vi "UnusedVI.vi"(9 "Queue in":refnum<queue>, 10 "queue in":refnum<queue>, 11 "String in":refnum<vi>) -> (3 "current sensor line ASCII":string)   [LabVIEW 2013]
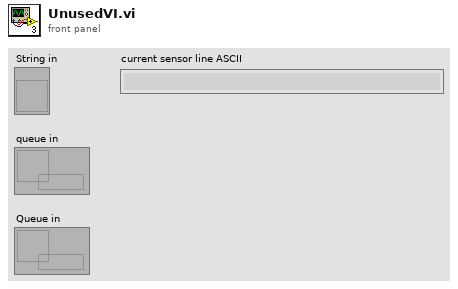
[diagram p1: front panel]
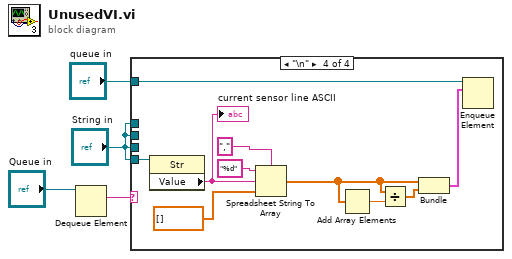
[diagram p0: block diagram]
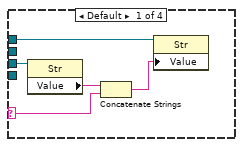
[diagram p2: hidden frame]
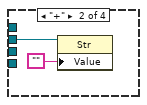
[diagram p3: hidden frame]
diagram:
  n1 = Dequeue Element(queue="Queue in") -> (element=w2:string)  [unwired: 2 in, 3 out]
  n2 = case shown="\"\\n\"" w2 {
    selector: w2 -> [w9 _ _ _]
    tunnel: "queue in" -> [_ _ _ w14]
    tunnel: "String in" -> [w6 _ _ _]
    tunnel: "String in" -> [w5 _ _ _]
    tunnel: "String in" -> [_ w10 _ _]
    tunnel: "String in" -> [_ _ _ w12]
    frame Default {
      n3 = property class="Str"(reference=w5) -> ("Value"=w7:string)  [unwired: 1 in, 2 out]
      n4 = Concatenate Strings(w7, w9) -> (w8:string)
      n5 = property class="Str"(reference=w6, "Value"=w8) -> ()  [unwired: 1 in, 2 out]
    }
    frame "+" {
      n6 = property class="Str"(reference=w10, "Value"="") -> ()  [unwired: 1 in, 2 out]
    }
    frame "\r" {
    }
    frame "\n" {
      n7 = property class="Str"(reference=w12) -> ("Value"=w17:string)  [unwired: 1 in, 2 out]
      "current sensor line ASCII" <- w17
      n8 = Spreadsheet String To Array(delimiter (Tab)=",", format string="%d", spreadsheet string=w17, array type (2D Dbl)=dbl[] []) -> (array=w15:dbl[])
      n9 = Add Array Elements(numeric array=w15) -> (sum=w18:dbl)
      n10 = Divide(x=w15, y=w18) -> (x/y=w16:dbl[])
      n11 = Bundle("array type (2D Dbl)"=w15, w16) -> (w13:cluster{"array type (2D Dbl)":dbl[], dbl[]})  [unwired: 1 in]
      n12 = Enqueue Element(queue=w14, element=w13) -> ()  [unwired: 2 in, 3 out]
    }
  }
